vi "SetCenter.vi"(8 "error in (no error)":errorcluster, 10 "center_position":T1, 11 "GameObject in":refnum<class "GameObject.lvclass">) -> (0 "error out":errorcluster, 3 "GameObject out":refnum<class "GameObject.lvclass">)   [LabVIEW 2019, in "RT_Game.lvlib" / "GameObject.lvclass"]
uses:
  GameObject.lvclass
  Game/Coordinate.ctl
  GameObject.lvclass/GameObject.ctl
  Game/Game.lvclass
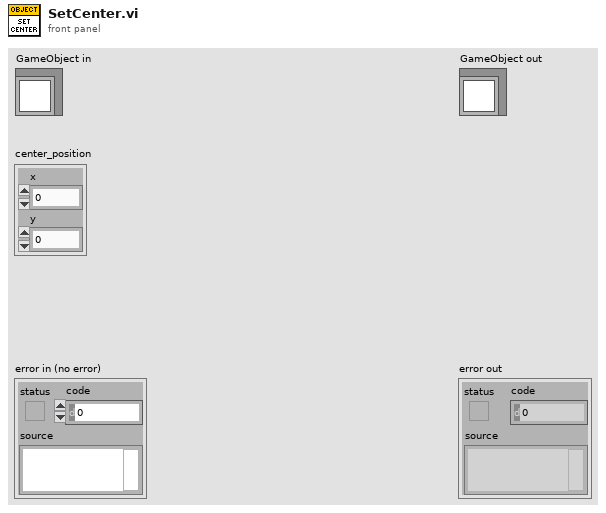
[diagram p1: front panel]
types:
  T1 = typedef "RT_Game.lvlib/Game.lvclass/Coordinate.ctl" = cluster{"x":dbl, "y":dbl}
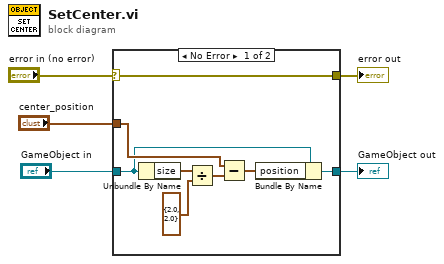
[diagram p0: block diagram]
diagram:
  n1 = case shown="No Error" "error in (no error)" {
    selector: "error in (no error)" -> [w13 w15]
    tunnel: [w13 w15] -> w4
    tunnel: [w9 w14] -> w2
    tunnel: "GameObject in" -> [w11 w14]
    tunnel: "center_position" -> [w12 _]
    frame No Error {
      n2 = Unbundle By Name(w11) -> ("size"=w10:T1)
      n3 = Divide(x=w10, y=T1 {"x"=2.0, "y"=2.0} ("x")) -> (x/y=w7:T1)
      n4 = Subtract(x=w12, y=w7) -> (x-y=w8:T1)
      n5 = Bundle By Name(cluster=w11, "position"=w8) -> (w9:refnum<class "GameObject.lvclass">)
    }
    frame Error {
    }
  }
  "error out" <- w4
  "GameObject out" <- w2
